vi "Apply Changes.vi"(8 "error in (no error)":errorcluster, 11 "New Project Wizard in":refnum<class "Update Project Wizard.lvclass">) -> (0 "error out":errorcluster, 3 "New Project Wizard out":refnum<class "Update Project Wizard.lvclass">)   [LabVIEW 2013, in "SET Project Editor.lvlib" / "Update Project Wizard.lvclass"]
uses:
  Update Project Wizard.lvclass
  UI Wizard/UI Wizard.lvclass
  <vilib>/ActorFramework/Actor/Actor.lvclass/Actor.ctl
  Update Project Wizard.lvclass/Update Project Wizard.ctl
  UI Wizard/UI Wizard.lvclass/UI Wizard.ctl
  <vilib>/ActorFramework/Message Enqueuer/Message Enqueuer.lvclass/Message Enqueuer.ctl
  UI Wizard/Read Project Data ref.vi
  <vilib>/ActorFramework/Message Enqueuer/Enqueue.vi
  <vilib>/ActorFramework/Message Priority Queue/Priority Enqueue.vi
  Controller Messages/Set Modified Flag Msg/Set Modified Flag Msg.lvclass
  Controller Messages/UI Refresh Msg/UI Refresh Msg.lvclass
  <vilib>/ActorFramework/Actor/Actor.lvclass
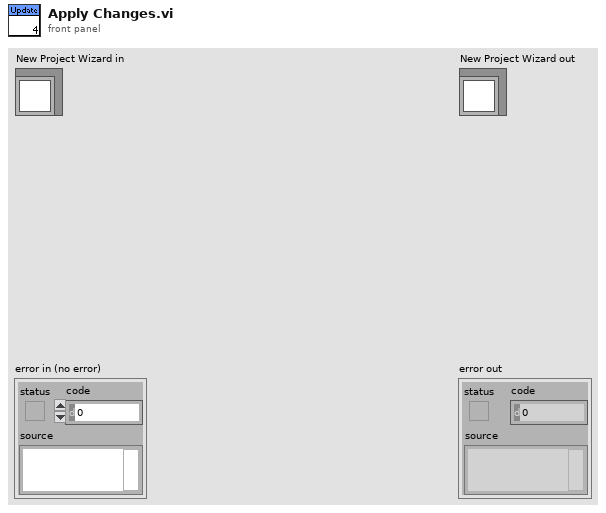
[diagram p1: front panel]
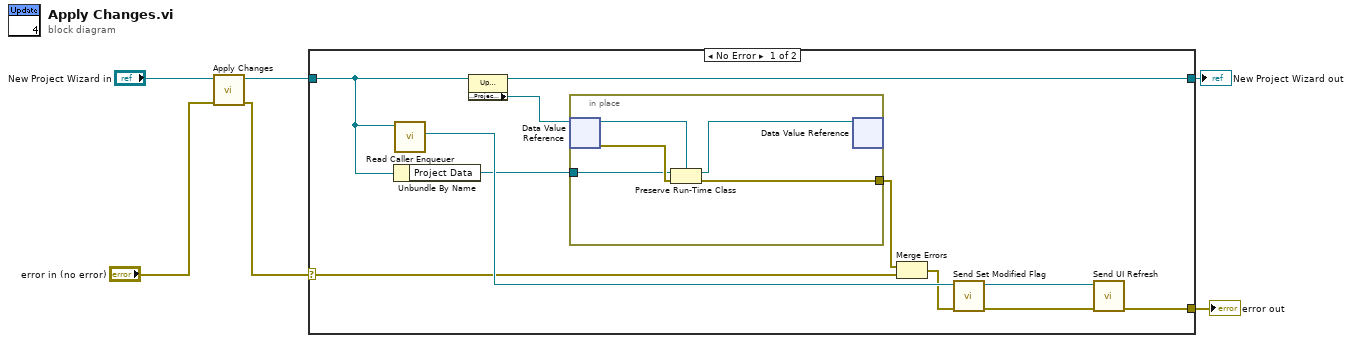
[diagram p0: block diagram]
diagram:
  n1 = call-parent "Apply Changes.vi"("error in (no error)"="error in (no error)", "UI Wizard in"="New Project Wizard in") -> ("error out"=w1:errorcluster, "UI Wizard out"=w4:refnum<class "Update Project Wizard.lvclass">)  [unwired: 8 in]
  n2 = case shown="No Error" w1 {
    selector: w1 -> [w8 w23]
    tunnel: w4 -> [w17 w24]
    tunnel: [w16 w24] -> w3
    tunnel: [w15 w23] -> w2
    frame No Error {
      n3 = Unbundle By Name(w17) -> ("Project Data"=w10:refnum<class "Project Data.lvclass">)
      n4 = call <vilib>:"Read Caller Enqueuer.vi"("Actor"=w17) -> ("Caller Enqueuer"=w13:refnum<class "Message Enqueuer.lvclass">)  [unwired: 10 in]
      n5 = property class="Update Project Wizard.lvclass"(reference=w17) -> (reference out=w16:refnum<class "Update Project Wizard.lvclass">, "Properties:Project Data ref"=w11:refnum<data-value>)  [unwired: 1 in, 1 out]
      n6 = in-place {
        in-place-border: w10 -> [w20]
        in-place-border: [w18] -> w9
        n7 = in-place-dvr #1(w11) -> (w22:refnum<class "Project Data.lvclass">, w21:errorcluster)
        n8 = Preserve Run-Time Class(object in=w20, error in=w21, 2:w22) -> (object out=w19:refnum<class "Project Data.lvclass">, error out=w18:errorcluster)
        n9 = in-place-dvr #1(w19) -> ()  [unwired: 2 out]
      }
      n10 = Merge Errors(w9, w8) -> (w7:errorcluster)
      n11 = call "Send Set Modified Flag.vi"("error in (no error)"=w7, "Message Enqueuer"=w13) -> ("error out"=w14:errorcluster, "Message Enqueuer out"=w12:refnum<class "Message Enqueuer.lvclass">)  [unwired: 8 in]
      n12 = call "Send UI Refresh.vi"("error in (no error)"=w14, "Message Enqueuer"=w12) -> ("error out"=w15:errorcluster)  [unwired: 8 in, 1 out]
    }
    frame Error {
    }
  }
  "error out" <- w2
  "New Project Wizard out" <- w3
